vi "write_serial.vi"(4 "error in (no error)":errorcluster, 6 "write buffer":string, 7 "VISA resource name":refnum<visa-resource-name>) -> (0 "error out":errorcluster, 2 "read buffer":string, 3 "VISA resource name out":refnum<visa-resource-name>)   [LabVIEW 2015]
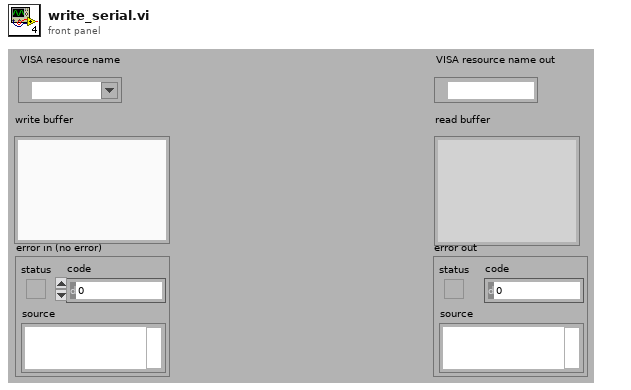
[diagram p1: front panel]
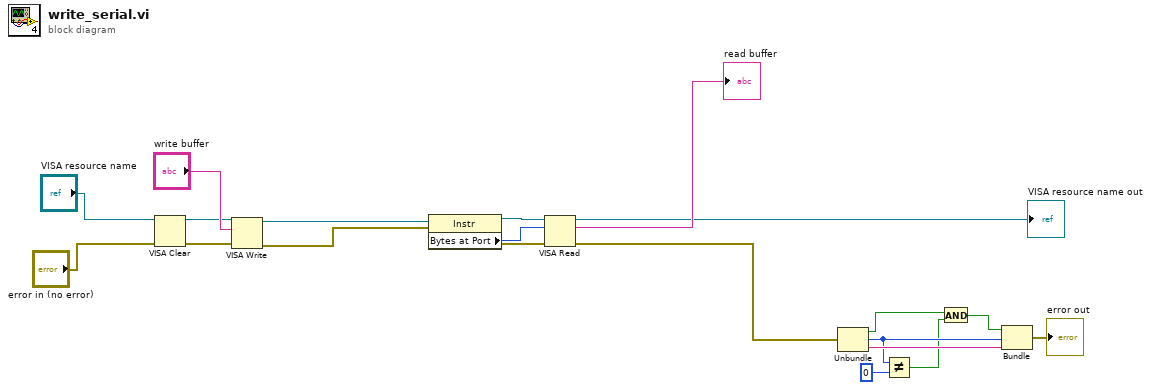
[diagram p0: block diagram]
diagram:
  n1 = VISA Clear(VISA resource name="VISA resource name", error in (no error)="error in (no error)") -> (VISA resource name out=w9:refnum<visa-resource-name>, error out=w8:errorcluster)
  n2 = VISA Write(VISA resource name=w9, write buffer="write buffer", error in (no error)=w8) -> (VISA resource name out=w12:refnum<visa-resource-name>, error out=w11:errorcluster)  [unwired: 1 out]
  n3 = property class="Instr"(reference=w12, error in=w11) -> (reference out=w4:refnum<visa-resource-name>, error out=w5:errorcluster, "Bytes at Port"=w3:u32)
  n4 = VISA Read(VISA resource name=w4, byte count=w3, error in (no error)=w5) -> (VISA resource name out=→"VISA resource name out":refnum<visa-resource-name>, read buffer=→"read buffer":string, error out=w1:errorcluster)  [unwired: 1 out]
  n5 = Unbundle(w1) -> ("status"=w10:bool, "code"=w16:i32, "source"=w18:string)
  n6 = Not Equal?(x=w16, y=0) -> (x != y?=w14:bool)
  n7 = And(x=w10, y=w14) -> (x .and. y?=w13:bool)
  n8 = Bundle(w13, "code"=w16, "source"=w18) -> (→"error out":cluster{bool, "code":i32, "source":string})  [unwired: 1 in]
